vi "update_zc_info5.vi"(6 "ywxinxi":string, 7 "status":string, 8 "didian":string, 9 "number":string, 10 "zerenren":string) -> (1 "data_str":string)   [LabVIEW 2017, in "Lib_code.lvlib"]
uses:
  Lib_code.lvlib
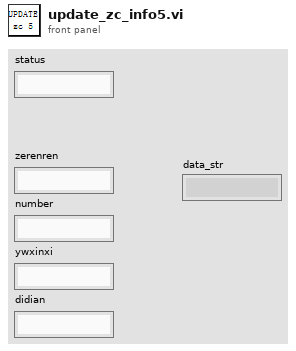
[diagram p1: front panel]
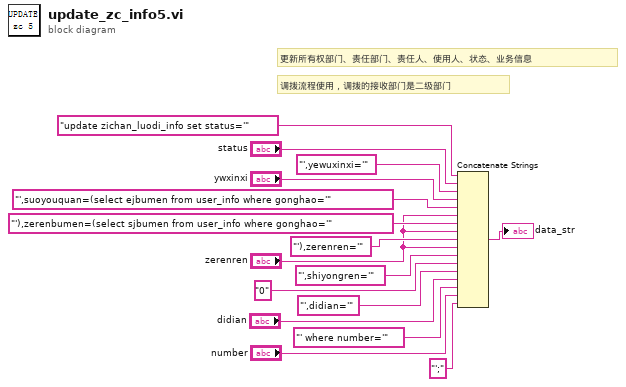
[diagram p0: block diagram]
diagram:
  # "调拨流程使用，调拨的接收部门是二级部门"
  # "更新所有权部门、责任部门、责任人、使用人、状态、业务信息"
  n1 = Concatenate Strings("update zichan_luodi_info set status='" ("Command Text"), "status", "',yewuxinxi='" ("字符串"), "ywxinxi", "',suoyouquan=(select ejbumen from user_info where gonghao='" ("字符串"), "zerenren", "'),zerenbumen=(select sjbumen from user_info where gonghao='" ("字符串"), "zerenren", "'),zerenren='" ("字符串"), "zerenren", "',shiyongren='" ("字符串"), "0" ("字符串"), "',didian='" ("字符串"), "didian", "' where number='" ("字符串"), "number", "';" ("字符串")) -> (→"data_str":string)
